vi "GSI-HVSwitch2.ProcPeriodic.vi"(0 "i ref in":refnum<vi>, 3 "ms timeout (10000)":i32=10000, 5 "error in (no error)":errorcluster) -> (14 "i ref out":refnum<vi>, 17 "timed out":bool, 19 "error out":errorcluster)   [LabVIEW 2014, in "GSI-HVSwitch2.lvlib"]
doc: "This method serves to periodically do things like reading values from the HW. Methods that should be executed periodically should be called from THIS method. Add code here.\n\nFor GSI-HVSwitch2 this method is not reentrant on purpose. The periodic action does the trending and should not block the system in case of lot's of GSI-HVSwitch2 devices."
uses:
  GSI-HVSwitch2.lvlib
  CSCore/CSApplicationBaseClasses/DeviceBase/DeviceBase.deviceState.ctl
  CSCore/CSObj/CSObj.lvlib
  CSCore/CSApplicationBaseClasses/DeviceBase/DeviceBase.lvlib
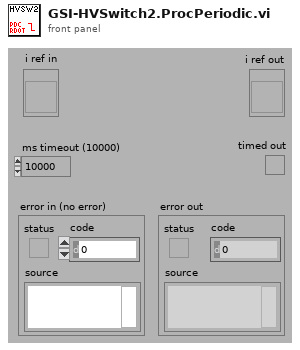
[diagram p1: front panel]
types:
  T1 = typedef "GSI-HVSwitch2.lvlib/GSI-HVSwitch2.i attribute.ctl" = cluster{"SDEX VISA Cluster":T2, "SetVoltage SW0":dbl, "SetVoltage SW1":dbl, "ActTempAmp":dbl, "ActTempPS1":dbl, "ActTempPS2":dbl, "mode":T5, "interfaceInitialized":bool, "serviceIDs":cluster{"nomVoltage0ID":i32, "nomVoltage1ID":i32, "actTempAmpID":i32, "actTempPS1ID":i32, "actTempPS2ID":i32, "modeID":i32}, "usedChannels":i32}
  T2 = typedef "SDEXDriver.lvlib/SDEX.VISA Control.ctl" = cluster{"VISA resource name":refnum<visa-resource-name>, "HEX address":u16, "VISA Timeout Value (1000 ms)":u32, "Lock Timeout (1000 ms)":u32, "semaphore":T3, "Baud rate":u32, "revision":T4, "deviceInfo":string}
  T3 = typedef "Semaphore RefNum" = refnum<k1>
  T4 = typedef "SDEXDriver.lvlib/SDEX.revisionType.ctl" = enum16{"unknown", "hvamp3", "hvswi1", "htrp0", "WDG0"}
  T5 = typedef "GSI-HVSwitch2.lvlib/GSI-HVSwitch2.mode.ctl" = enum16{"unknown", "switch", "stepper"}
  T6 = typedef "DeviceBase.lvlib/DeviceBase.deviceState.ctl" = i16
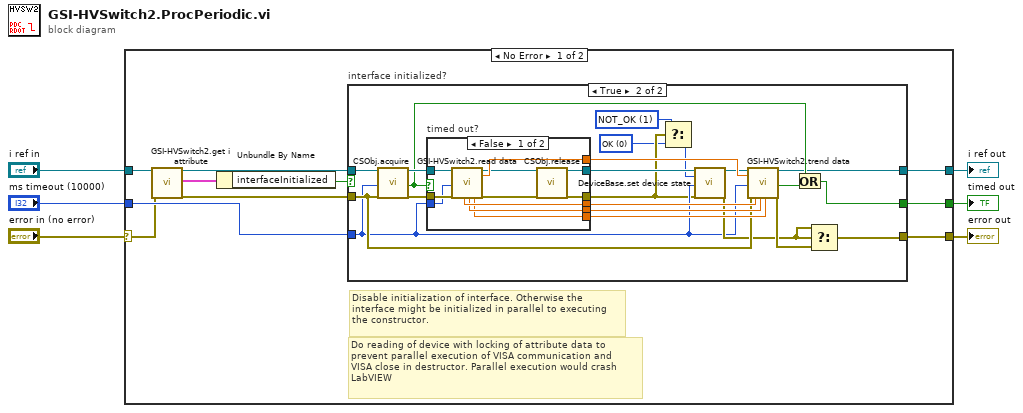
[diagram p0: block diagram]
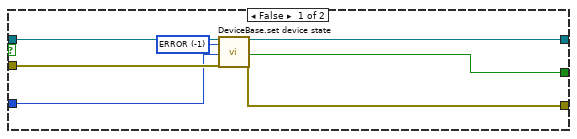
[diagram p2: hidden frame]
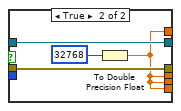
[diagram p3: hidden frame]
diagram:
  n1 = case shown="No Error" "error in (no error)" {
    selector: "error in (no error)" -> [w10 w61]
    tunnel: "ms timeout (10000)" -> [w16 _]
    tunnel: [w9 w62] -> w5
    tunnel: [w15 w61] -> w4
    tunnel: "i ref in" -> [w14 w62]
    tunnel: [w7 _] -> w2
    frame No Error {
      # "Do reading of device with locking of attribute data to\nprevent parallel execution of VISA communication and \nVISA close in destructor. Parallel execution would crash\nLabVIEW"
      # "Disable initialization of interface. Otherwise the\ninterface might be initialized in parallel to executing\nthe constructor."
      n2 = call "GSI-HVSwitch2.get i attribute.vi"("i ref in"=w14, "error in (no error)"=w10) -> ("i ref out"=w12:refnum<vi>, "i attribute"=w11:T1, "error out"=w13:errorcluster)  [unwired: 15 in]
      n3 = Unbundle By Name(w11) -> ("interfaceInitialized"=w8:bool)
      n4 = case "interface initialized?" shown="True" w8 {
        tunnel: w16 -> [w18 w28]
        tunnel: [w22 w32] -> w9
        tunnel: [w20 w41] -> w15
        tunnel: w13 -> [w21 w36]
        tunnel: w12 -> [w23 w39]
        tunnel: [w17 w35] -> w7
        frame False {
          w19 = T6 -1 items=["ERROR"=-1, "OK"=0, "NOT_OK"=1] ("deviceState")
          n5 = call "DeviceBase.set device state.vi"("i ref in"=w23, "deviceState"=w19, "ms timeout (10000)"=w18, "error in (no error)"=w21) -> ("i ref out"=w22:refnum<vi>, "timed out"=w17:bool, "error out"=w20:errorcluster)  [unwired: 13 in]
        }
        frame True {
          w24 = T6 1 items=["ERROR"=-1, "OK"=0, "NOT_OK"=1] ("deviceState")
          w26 = T6 0 items=["ERROR"=-1, "OK"=0, "NOT_OK"=1] ("deviceState")
          n6 = call "CSObj.acquire.vi"("i ref in"=w39, "ms timeout (10000)"=w28, "error in (no error)"=w36) -> ("i ref out"=w38:refnum<vi>, "timed out"=w34:bool, "error out"=w37:errorcluster)  [unwired: 14 in]
          n7 = case "timed out?" shown="False" w34 {
            tunnel: [w48 w59] -> w31
            tunnel: [w56 w57] -> w45
            tunnel: [w55 w57] -> w44
            tunnel: [w54 w57] -> w43
            tunnel: [w53 w57] -> w42
            tunnel: [w46 w58] -> w27
            tunnel: w37 -> [w52 w58]
            tunnel: w28 -> [w51 _]
            tunnel: w38 -> [w50 w59]
            frame False {
              n8 = call "GSI-HVSwitch2.read data.vi"("i ref in"=w50, "ms timeout (10000)"=w51, "error in (no error)"=w52) -> ("ActTempAmp"=w55:dbl, "ActTempPS1"=w54:dbl, "ActTempPS2"=w53:dbl, "i ref out"=w49:refnum<vi>, "ActVoltage"=w56:dbl, "error out"=w47:errorcluster)  [unwired: 10 in, 1 out]
              n9 = call "CSObj.release.vi"("i ref in"=w49, "error in (no error)"=w47) -> ("i ref out"=w48:refnum<vi>, "error out"=w46:errorcluster)  [unwired: 16 in]
            }
            frame True {
              n10 = To Double Precision Float(number=u16 32768) -> (double precision float=w57:dbl)
            }
          }
          n11 = Select(t=w24, s=w27, f=w26) -> (s? t:f=w25:T6)
          n12 = call "DeviceBase.set device state.vi"("i ref in"=w31, "deviceState"=w25, "ms timeout (10000)"=w28, "error in (no error)"=w27) -> ("i ref out"=w30:refnum<vi>, "error out"=w29:errorcluster)  [unwired: 13 in, 1 out]
          n13 = call "GSI-HVSwitch2.trend data.vi"("i ref in"=w30, "ActVoltage"=w45, "ms timeout (10000)"=w28, "error in (no error)"=w36, "ActTempAmp"=w44, "ActTempPS1"=w43, "ActTempPS2"=w42) -> ("i ref out"=w32:refnum<vi>, "timed out"=w33:bool, "error out"=w40:errorcluster)  [unwired: 10 in]
          n14 = Or(x=w34, y=w33) -> (x .or. y?=w35:bool)
          n15 = Select(t=w29, s=w29, f=w40) -> (s? t:f=w41:errorcluster)
        }
      }
    }
    frame Error {
    }
  }
  "error out" <- w4
  "i ref out" <- w5
  "timed out" <- w2
